vi "Destroy Broadcast Events.vi"(8 "error in":errorcluster) -> (0 "error out":errorcluster)   [LabVIEW 2021, in "Sequence Engine.lvlib"]
doc: "Destroy the broadcast events, even if there is an incoming error.\n\n<b>NOTE</b>: The contents of this VI are automatically generated and modified by the <b>Tools > DQMH Consortium > DQMH</b> utilities. Consider using those utilities instead of making your own modifications to this VI.\n_____\nBased on DQMH Dev Tools: Project Template 7.1.1.1528."
uses:
  Sequence Engine.lvlib
panel:
  # "NOTE: The contents of this VI are automatically generated and modified by the Tools > DQMH Consortium > DQMH utilities. Consider using those utilities instead of making your own modifications to this VI."
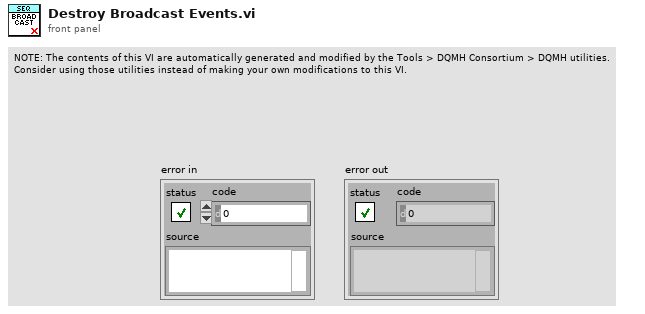
[diagram p1: front panel]
types:
  T1 = typedef "Sequence Engine.lvlib/Broadcast Events--cluster.ctl" = cluster{"Module Did Init":refnum<user-event>, "Status Updated":refnum<user-event>, "Error Reported":refnum<user-event>, "Module Did Stop":refnum<user-event>, "Update Module Execution Status":refnum<user-event>, "New Test Result":refnum<user-event>, "Testing Started":refnum<user-event>, "Testing Completed":refnum<user-event>, "Retried Count":refnum<user-event>, "DUT Info":refnum<user-event>, "Stop Testing":refnum<user-event>}
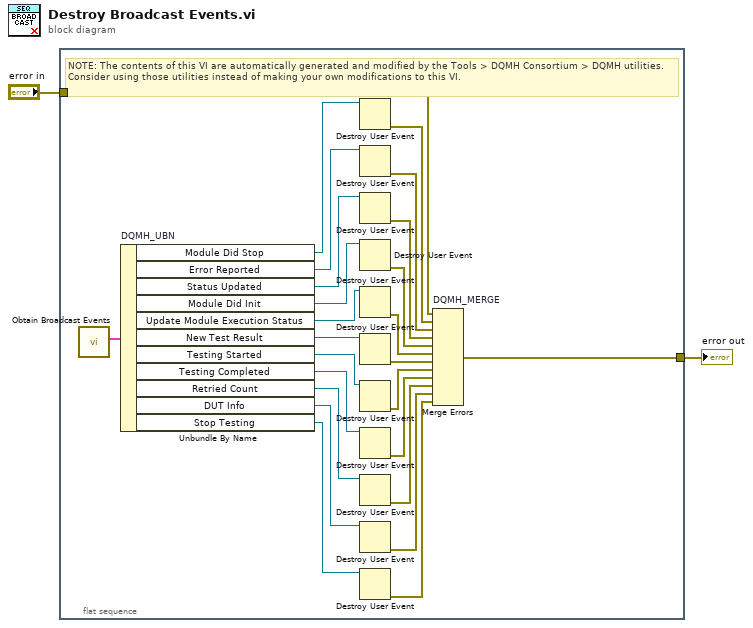
[diagram p0: block diagram]
diagram:
  n1 = flat-sequence {
    tunnel: [w26] -> w2
    tunnel: "error in" -> [w17]
    frame #0 {
      # "NOTE: The contents of this VI are automatically generated and modified by the Tools > DQMH Consortium > DQMH utilities. Consider using those utilities instead of making your own modifications to this VI."
      n2 = call "Obtain Broadcast Events.vi"() -> ("Sequence Engine Broadcast Events"=w25:T1)  [unwired: 10 in, 1 out]
      n3 = Unbundle By Name "DQMH_UBN"(w25) -> ("Module Did Stop"=w18:refnum<user-event>, "Error Reported"=w20:refnum<user-event>, "Status Updated"=w23:refnum<user-event>, "Module Did Init"=w24:refnum<user-event>, "Update Module Execution Status"=w15:refnum<user-event>, "New Test Result"=w13:refnum<user-event>, "Testing Started"=w11:refnum<user-event>, "Testing Completed"=w9:refnum<user-event>, "Retried Count"=w7:refnum<user-event>, "DUT Info"=w5:refnum<user-event>, "Stop Testing"=w3:refnum<user-event>)
      n4 = Destroy User Event(user event=w18) -> (error out=w19:errorcluster)  [unwired: 1 in]
      n5 = Destroy User Event(user event=w20) -> (error out=w21:errorcluster)  [unwired: 1 in]
      n6 = Destroy User Event(user event=w23) -> (error out=w22:errorcluster)  [unwired: 1 in]
      n7 = Destroy User Event(user event=w24) -> (error out=w27:errorcluster)  [unwired: 1 in]
      n8 = Destroy User Event(user event=w15) -> (error out=w16:errorcluster)  [unwired: 1 in]
      n9 = Destroy User Event(user event=w13) -> (error out=w14:errorcluster)  [unwired: 1 in]
      n10 = Destroy User Event(user event=w11) -> (error out=w12:errorcluster)  [unwired: 1 in]
      n11 = Destroy User Event(user event=w9) -> (error out=w10:errorcluster)  [unwired: 1 in]
      n12 = Destroy User Event(user event=w7) -> (error out=w8:errorcluster)  [unwired: 1 in]
      n13 = Destroy User Event(user event=w5) -> (error out=w6:errorcluster)  [unwired: 1 in]
      n14 = Destroy User Event(user event=w3) -> (error out=w4:errorcluster)  [unwired: 1 in]
      n15 = Merge Errors "DQMH_MERGE"(w17, w19, w21, w22, w27, w16, w14, w12, w10, w8, w6, w4) -> (w26:errorcluster)
    }
  }
  "error out" <- w2
